vi "zmq_getsocketopt_binary.vi"(3 "error in":errorcluster, 4 "option":T1=enum."ZMQ_SWAP", 5 "socket in":refnum<class "zmq_socket.lvclass">) -> (0 "error out":errorcluster, 1 "value":string, 2 "socket out":refnum<class "zmq_socket.lvclass">)   [LabVIEW 2020, in "zeromq.lvlib" / "zmq_socket.lvclass"]
doc: "Query the value of <b>option</b> for the given <b>socket</b>.\n\nYou are responsible for selecting the correct polymorphic instance for the option you wish to query. Valid options of the binary type are: ZMQ_IDENTITY\n\nFurther API documentation: http://api.zeromq.org/3-2:zmq-getsockopt"
uses:
  zmq_socket.lvclass
  socket_options.ctl
  zmq_socket.lvclass/zmq_socket.ctl
  zeromq.lvlib
panel:
  out "len":u32
  # "ØMQ"
  # "labview"
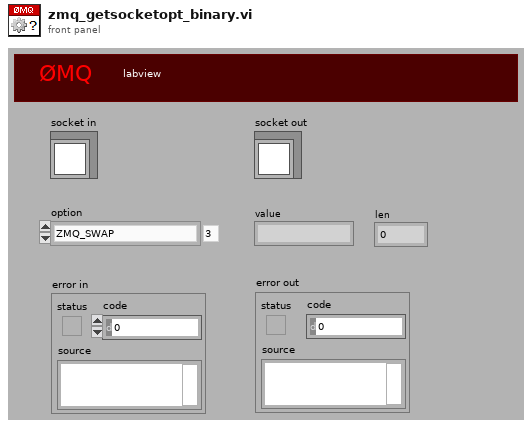
[diagram p1: front panel]
types:
  T1 = typedef "zeromq.lvlib/socket_options.ctl" = enum8{"NONE", "ZMQ_HWM", "<2>", "ZMQ_SWAP", "ZMQ_AFFINITY", "ZMQ_IDENTITY", "ZMQ_SUBSCRIBE", "ZMQ_UNSUBSCRIBE", "ZMQ_RATE", "ZMQ_RECOVERY_IVL", "ZMQ_MCAST_LOOP", "ZMQ_SNDBUF", "ZMQ_RCVBUF", "ZMQ_RCVMORE", "ZMQ_FD", "ZMQ_EVENTS", "ZMQ_TYPE", "ZMQ_LINGER", "ZMQ_RECONNECT_IVL", "ZMQ_BACKLOG", "ZMQ_RECOVERY_IVL_MSEC", "ZMQ_RECONNECT_IVL_MAX", "ZMQ_MAXMSGSIZE", "ZMQ_SNDHWM", "ZMQ_RCVHWM", "ZMQ_MULTICAST_HOPS", "<26>", "ZMQ_RCVTIMEO", "ZMQ_SNDTIMEO", "<29>", "<30>", "ZMQ_IPV4ONLY", "ZMQ_LAST_ENDPOINT", "ZMQ_ROUTER_MANDATORY", "ZMQ_TCP_KEEPALIVE", "ZMQ_TCP_KEEPALIVE_CNT", "ZMQ_TCP_KEEPALIVE_IDLE", "ZMQ_TCP_KEEPALIVE_INTVL", "ZMQ_TCP_ACCEPT_FILTER", "ZMQ_DELAY_ATTACH_ON_CONNECT", "ZMQ_XPUB_VERBOSE"}
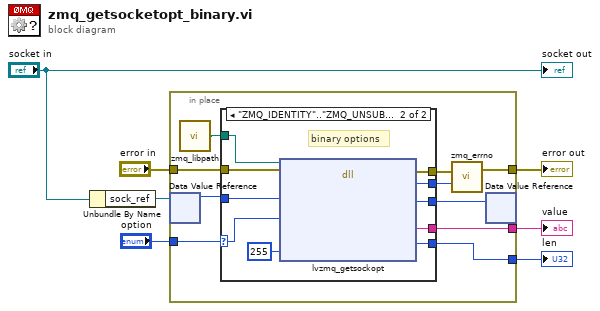
[diagram p0: block diagram]
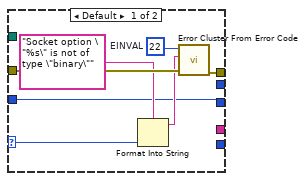
[diagram p2: hidden frame]
diagram:
  n1 = Unbundle By Name("socket in") -> ("sock_ref"=w1:refnum<data-value>)
  n2 = in-place {
    in-place-border: [w15] -> w7
    in-place-border: "error in" -> [w14]
    in-place-border: "option" -> [w13]
    in-place-border: [w12] -> w4
    in-place-border: [w11] -> w3
    n3 = in-place-dvr #1(w1) -> (w10:u64)  [unwired: 1 out]
    n4 = call "zmq_libpath.vi"() -> ("path"=w8:path)
    n5 = case shown="\"ZMQ_IDENTITY\"..\"ZMQ_UNSUBSCRIBE\", \"ZMQ_LAST_ENDPOINT\"" w13 {
      selector: w13 -> [w21 w32]
      tunnel: [w24 w34] -> w17
      tunnel: [_ w33] -> w16
      tunnel: w14 -> [w22 w30]
      tunnel: [_ w29] -> w12
      tunnel: [_ w28] -> w11
      tunnel: w10 -> [w18 w27]
      tunnel: [w18 w26] -> w9
      tunnel: w8 -> [_ w25]
      frame Default {
        w23 = 22  # EINVAL
        n6 = Format Into String(format string="Socket option \"%s\" is not of type \"binary\"", w21) -> (resulting string=w19:string)  [unwired: 2 in, 1 out]
        n7 = call "Error Cluster From Error Code.vi"("error in (no error)"=w22, "error message (\"\")"=w19, "error code (0)"=w23) -> ("error out"=w24:errorcluster)  [unwired: 6 in]
      }
      frame "ZMQ_IDENTITY".."ZMQ_UNSUBSCRIBE", "ZMQ_LAST_ENDPOINT" {
        # "binary options"
        n8 = dll-call lib="?" fn="lvzmq_getsockopt"(path in=w25, error in=w30, "socket"=w27, "option"=w32, "len"=u32 255) -> (error out=w34:errorcluster, "return type"=w33:i32, "socket"=w26:u64, "data"=w29:string, "len"=w28:u32)  [unwired: 3 in, 1 out]
      }
    }
    n9 = call "zmq_errno.vi"("retval"=w16, "error in"=w17) -> ("error out"=w15:errorcluster)  [unwired: 1 out]
    n10 = in-place-dvr #1(w9) -> ()  [unwired: 2 out]
  }
  "error out" <- w7
  "value" <- w4
  "len" <- w3
  "socket out" <- "socket in"
